vi "Update Listeners.vi"(8 "error in":errorcluster, 11 "Data Subject in":refnum<class "Data Subject.lvclass">) -> (0 "error out":errorcluster, 3 "Data Subject out":refnum<class "Data Subject.lvclass">)   [LabVIEW 2018, in "Data Subject.lvclass"]
uses:
  Data Subject.lvclass
  Data/Data.lvclass
  Data Subject.lvclass/Data Subject.ctl
panel:
  in  "DVR":refnum<data-value>
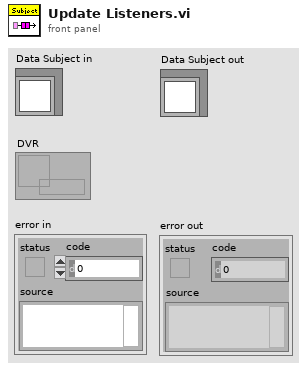
[diagram p1: front panel]
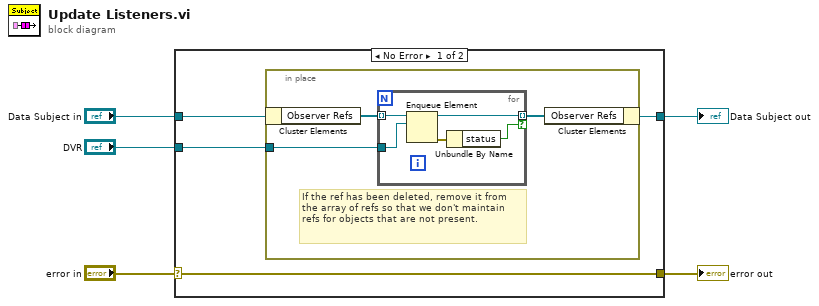
[diagram p0: block diagram]
diagram:
  n1 = case shown="No Error" "error in" {
    selector: "error in" -> [w9 w19]
    tunnel: [w9 w19] -> w4
    tunnel: [w6 w18] -> w2
    tunnel: "Data Subject in" -> [w7 w18]
    tunnel: "DVR" -> [w8 _]
    frame No Error {
      n2 = in-place {
        in-place-border: w8 -> [w12]
        # "If the ref has been deleted, remove it from the array of refs so that we don't maintain refs for objects that are not present."
        n3 = in-place-cluster #1(w7) -> ("Observer Refs"=w11:refnum<queue>[])
        n4 = for {
          tunnel: [w17] -> w10 mode=indexing if=w15
          tunnel: w12 -> [w14]
          tunnel: w11 -> [w13] mode=indexing
          n5 = Enqueue Element(queue=w13, element=w14) -> (queue out=w17:refnum<queue>, error out=w16:errorcluster)  [unwired: 2 in, 1 out]
          n6 = Unbundle By Name(w16) -> ("status"=w15:bool)
        }
        n7 = in-place-cluster #1("Observer Refs"=w10) -> (w6:refnum<class "Data Subject.lvclass">)
      }
    }
    frame Error {
    }
  }
  "error out" <- w4
  "Data Subject out" <- w2
